vi "Gestione nomi utenti.vi"(3 "Message":string, 8 "error in (no error)":errorcluster, 11 "name or relative path":string="Settings\\utenti.txt") -> (0 "error out":errorcluster, 2 "Utenti Read":string[][](array[string]))   [LabVIEW 2019]
uses:
  <vilib>/Utility/file.llb/Read Delimited Spreadsheet (string).vi
  <vilib>/Utility/file.llb/Write Delimited Spreadsheet (string).vi
panel:
  in  "Utenti":string[][](array[string])
  in  "Exit":bool
  in  "Write file":bool
  in  "Read file":bool
  # "Position"
  # "Nomi"
  # "Position"
  # "Nomi"
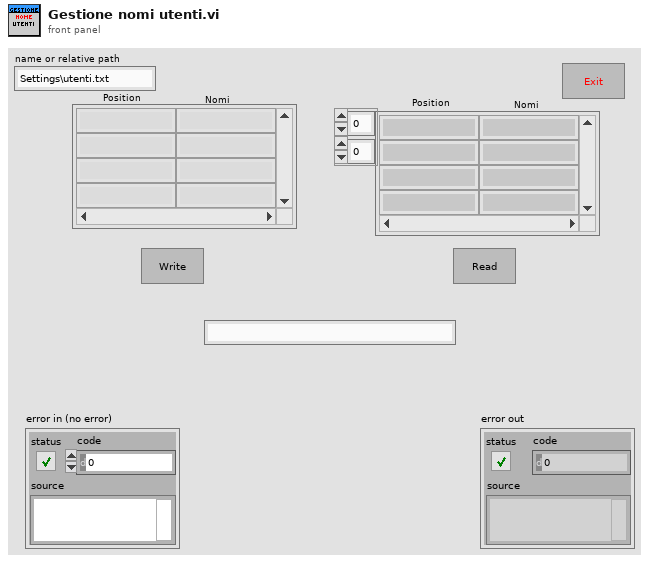
[diagram p1: front panel]
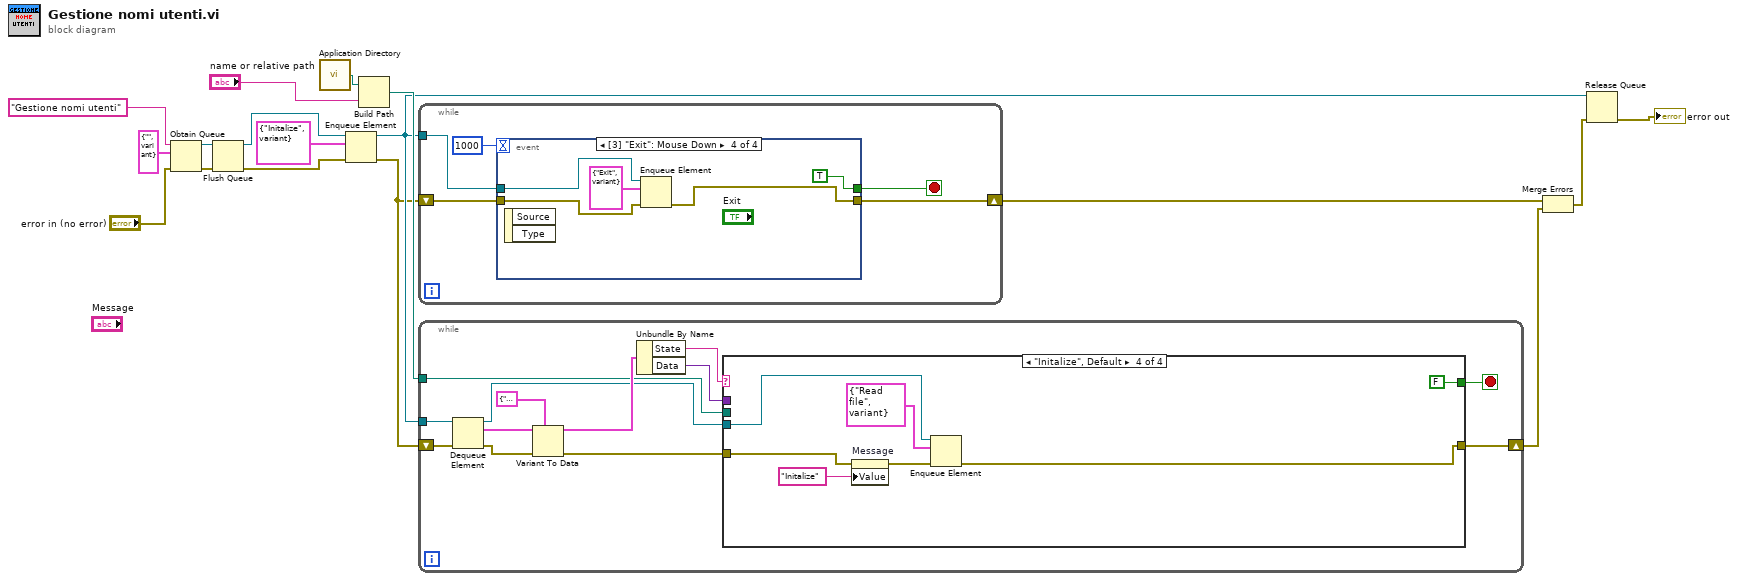
[diagram p0: block diagram]
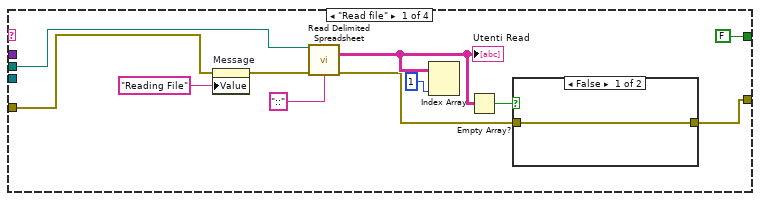
[diagram p2: hidden frame]
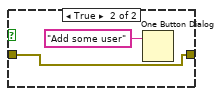
[diagram p3: hidden frame]
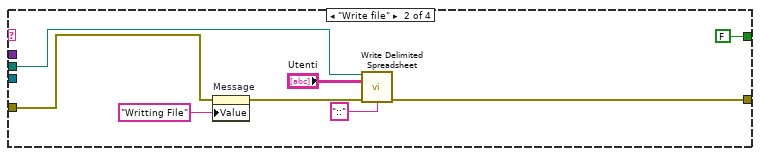
[diagram p4: hidden frame]
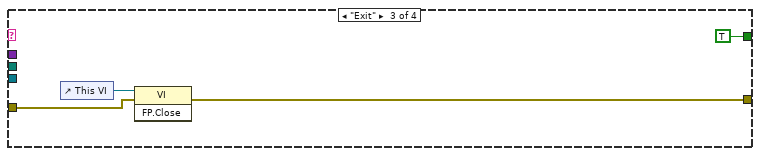
[diagram p5: hidden frame]
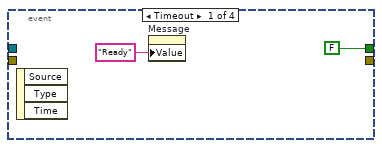
[diagram p6: hidden frame]
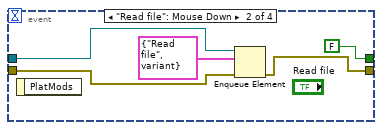
[diagram p7: hidden frame]
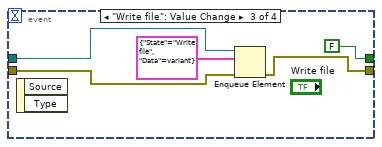
[diagram p8: hidden frame]
diagram:
  n1 = Obtain Queue(name (unnamed)="Gestione nomi utenti", element data type=cluster{"State":string, "Data":variant} {"State"="", "Data"=variant}, error in (no error)="error in (no error)") -> (queue out=w17:refnum<queue>, error out=w16:errorcluster)  [unwired: 2 in, 1 out]
  n2 = Flush Queue(queue=w17, error in (no error)=w16) -> (queue out=w15:refnum<queue>, error out=w14:errorcluster)  [unwired: 1 out]
  n3 = call <vilib>:"Application Directory.vi"() -> ("Application Directory"=w10:path)
  n4 = Enqueue Element(queue=w15, element=cluster{"State":string, "Data":variant} {"State"="Initalize", "Data"=variant}, error in (no error)=w14) -> (queue out=w7:refnum<queue>, error out=w6:errorcluster)  [unwired: 1 in, 1 out]
  n5 = Build Path(base path=w10, name or relative path="name or relative path") -> (appended path=w8:path)
  n6 = while {
    tunnel: w7 -> [w22]
    shift-right: [w18] -> w4
    shift-left: w6 -> [w19]
    stop <- w20 stop-if-true
    n7 = event shown="[3] \"Exit\": Mouse Down" {
      selector: _ -> [_ _ _ _]
      dyn-events: _ -> [_ _ _ _]
      timeout: 1000 -> [_ _ _ _]
      tunnel: w22 -> [_ w28 w33 w37]
      tunnel: [FALSE FALSE FALSE TRUE] -> w20
      tunnel: [_ w26 w30 w35] -> w18
      tunnel: w19 -> [_ w25 w31 w36]
      event Timeout {
        n8 = event-data() -> ()  [unwired: 1 in, 3 out]
        n9 = property on="Message" class="Str"("Value"="Ready" ("Message")) -> ()  [unwired: 2 in, 2 out]
      }
      event "Read file": Mouse Down {
        n10 = event-data() -> ()  [unwired: 1 in, 1 out]
        n11 = Enqueue Element(queue=w28, element=cluster{"State":string, "Data":variant} {"State"="Read file", "Data"=variant}, error in (no error)=w25) -> (error out=w26:errorcluster)  [unwired: 1 in, 2 out]
      }
      event "Write file": Value Change {
        n12 = event-data() -> ()  [unwired: 1 in, 2 out]
        n13 = Enqueue Element(queue=w33, element=cluster{"State":string, "Data":variant} {"State"="Write file", "Data"=variant}, error in (no error)=w31) -> (error out=w30:errorcluster)  [unwired: 1 in, 2 out]
      }
      event "Exit": Mouse Down {
        n14 = event-data() -> ()  [unwired: 1 in, 2 out]
        n15 = Enqueue Element(queue=w37, element=cluster{"State":string, "Data":variant} {"State"="Exit", "Data"=variant}, error in (no error)=w36) -> (error out=w35:errorcluster)  [unwired: 1 in, 2 out]
      }
    }
  }
  n16 = while {
    tunnel: w7 -> [w52]
    tunnel: w8 -> [w44]
    shift-right: [w40] -> w5
    shift-left: w6 -> [w51]
    stop <- w41 stop-if-true
    n17 = Dequeue Element(queue=w52, error in (no error)=w51) -> (queue out=w43:refnum<queue>, element=w49:cluster{"State":string, "Data":variant}, error out=w50:errorcluster)  [unwired: 1 in, 1 out]
    n18 = Variant To Data(error in=w50, type=cluster{"State":string, "Data":variant} {"State"="", "Data"=variant}, Variant=w49) -> (data=w47:cluster{"State":string, "Data":variant}, error out=w42:errorcluster)
    n19 = Unbundle By Name(w47) -> ("State"=w46:string, "Data"=w45:variant)
    n20 = case shown="\"Initalize\", Default" w46 {
      tunnel: w45 -> [_ _ _ _]
      tunnel: w44 -> [w62 w74 _ _]
      tunnel: w43 -> [_ _ _ w85]
      tunnel: w42 -> [w56 w69 w76 w81]
      tunnel: [FALSE FALSE TRUE FALSE] -> w41
      tunnel: [w53 w67 w75 w79] -> w40
      frame "Read file" {
        n21 = property on="Message" class="Str"(error in=w56, "Value"="Reading File" ("Message")) -> (error out=w55:errorcluster)  [unwired: 1 in, 1 out]
        n22 = call-poly <vilib>:"Read Delimited Spreadsheet.vi"("file path (dialog if empty)"=w62, "error in (no error)"=w55, "delimiter (\\t)"="::" ("delimiter (\\t)")) -> ("all rows"=w61:string[][], "error out"=w54:errorcluster)  [unwired: 7 in, 4 out]
        "Utenti Read" <- w61
        n23 = Index Array(array=w61, index (col)=1 ("disabled index (col)")) -> ()  [unwired: 1 in, 1 out]
        n24 = Empty Array?(array=w61) -> (empty?=w60:bool)
        n25 = case shown="False" w60 {
          tunnel: w54 -> [w64 w65]
          tunnel: [w64 w65] -> w53
          frame False {
          }
          frame True {
            n26 = One Button Dialog(message="Add some user") -> ()  [unwired: 1 in, 1 out]
          }
        }
      }
      frame "Write file" {
        n27 = property on="Message" class="Str"(error in=w69, "Value"="Writting File" ("Message")) -> (error out=w68:errorcluster)  [unwired: 1 in, 1 out]
        n28 = call-poly <vilib>:"Write Delimited Spreadsheet.vi"("file path (dialog if empty)"=w74, "2D data"="Utenti", "error in (no error)"=w68, "delimiter (\\t)"="::" ("delimiter (\\t)")) -> ("error out"=w67:errorcluster)  [unwired: 10 in, 1 out]
      }
      frame "Exit" {
        n29 = control-ref of="This VI"() -> (w78:refnum<vi>)
        n30 = invoke class="VI" method="FP.Close"(reference=w78, error in=w76) -> (error out=w75:errorcluster)  [unwired: 1 in, 2 out]
      }
      frame "Initalize", Default {
        n31 = property on="Message" class="Str"(error in=w81, "Value"="Initalize" ("Message")) -> (error out=w80:errorcluster)  [unwired: 1 in, 1 out]
        n32 = Enqueue Element(queue=w85, element=cluster{"State":string, "Data":variant} {"State"="Read file", "Data"=variant}, error in (no error)=w80) -> (error out=w79:errorcluster)  [unwired: 1 in, 2 out]
      }
    }
  }
  n33 = Merge Errors(w4, w5) -> (w3:errorcluster)
  n34 = Release Queue(queue=w7, error in (no error)=w3) -> (error out=→"error out":errorcluster)  [unwired: 1 in, 2 out]
